vi "New Edit Element.vi"(8 "error in (no error)":errorcluster, 11 "_ISerializable in":refnum<class "_ISerializable.lvclass">) -> (0 "error out":errorcluster, 3 "_ISerializable out":refnum<class "_ISerializable.lvclass">)   [LabVIEW 2018, in "_ISerializable.lvclass"]
uses:
  _ISerializable.lvclass
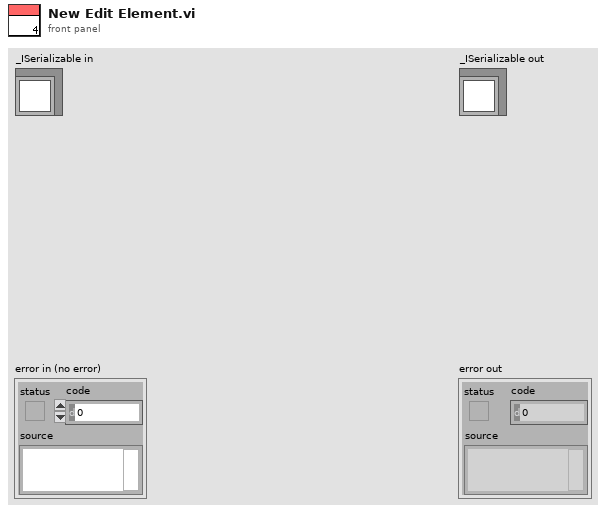
[diagram p1: front panel]
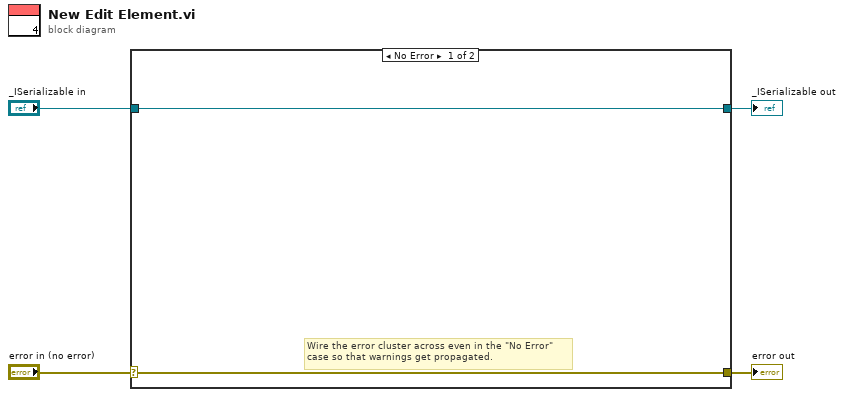
[diagram p0: block diagram]
diagram:
  n1 = case shown="No Error" "error in (no error)" {
    selector: "error in (no error)" -> [w5 w8]
    tunnel: [w5 w8] -> w3
    tunnel: [w6 w7] -> w1
    tunnel: "_ISerializable in" -> [w6 w7]
    frame No Error {
      # "Wire the error cluster across even in the \"No Error\"\ncase so that warnings get propagated."
    }
    frame Error {
    }
  }
  "error out" <- w3
  "_ISerializable out" <- w1
